vi "SC_schleife_init_20TVTI.vi"   [LabVIEW 2019]
uses:
  Monitors/Utility/Monitor Communication/Gustav/20TVTI_Control.ctl
  Global/Global Variables/global.vi
  Instrument_Setup.vi
  Global/Global Variables/Data_Display_global.vi
types:
  T1 = typedef "20TVTI_Cluster.ctl" = cluster{"Temperatur (K)":dbl, "Setpoint (K)":dbl, "Rate (K/min)":dbl, "Heater (%)":dbl, "NV (%)":dbl, "Heater Manual":bool, "NV Manual":bool, "Go to Set":bool, "Heater SP":dbl, "Valid?":bool, "Set Heater SP":bool, "Set NV SP":bool, "Heater (%) Display":dbl, "NV (%) Display":dbl, "NV Setpoint":dbl, "Change Heater Status":bool, "Change NV Status":bool, "Stop":bool, "Current T Setpoint":dbl, "Sweeping?":bool, "Sweep Mode":string, "Change Sweep Mode":bool}
  T2 = typedef "20TVTI_Control.ctl" = cluster{"Set VTI SP":bool, "Change NV Status":bool, "Set NV Setpoint":bool, "Change Heater Status":bool, "Set Heater Setpoint":bool, "Stop Sweep":bool, "Setpoint (K)":dbl, "Rate (K/min)":dbl, "Setpoint Heater":dbl, "Setpoint NV":dbl, "Change Sweep Mode":bool}
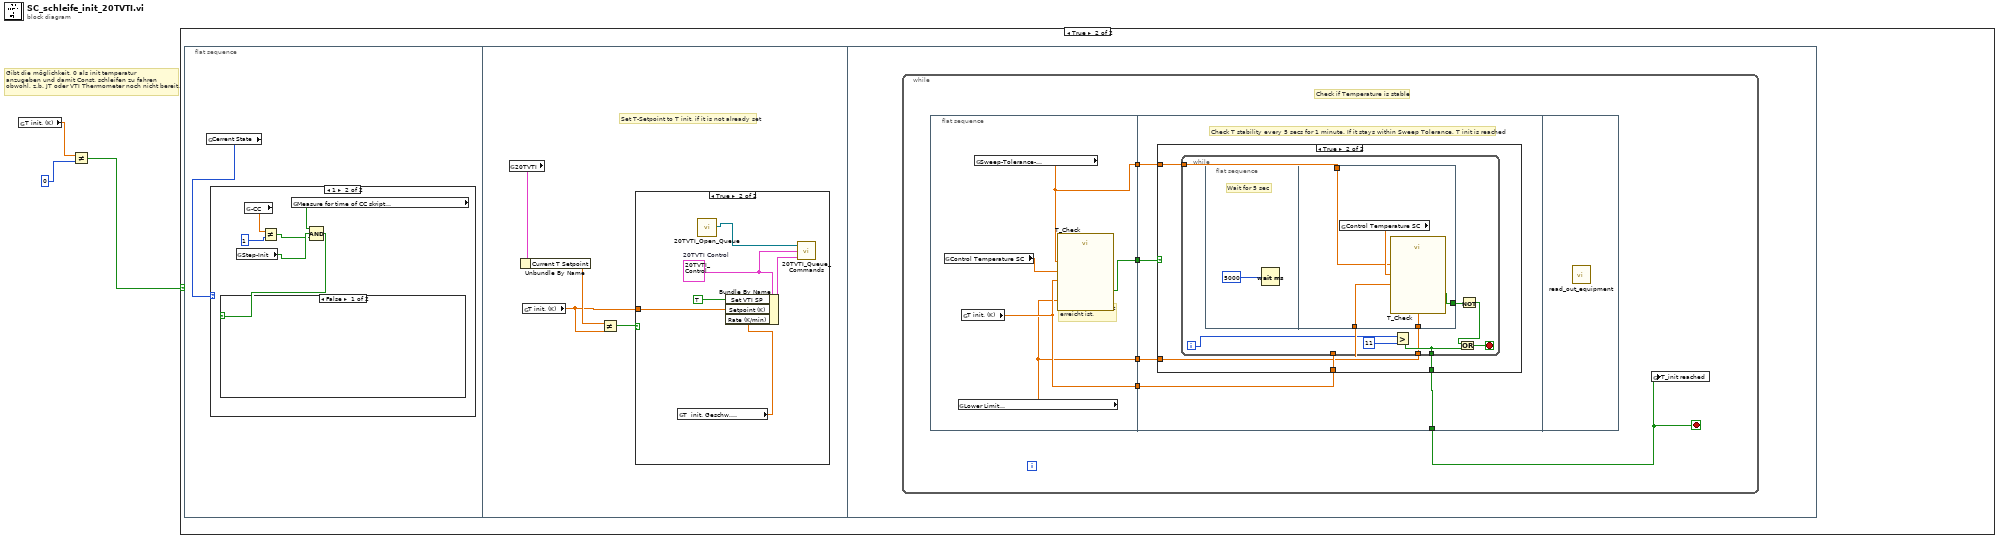
[diagram p0: block diagram]
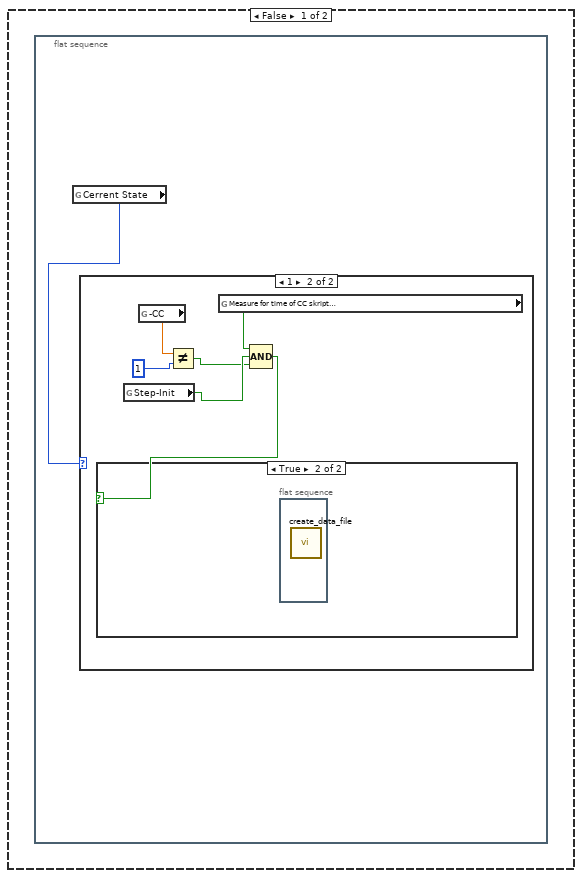
[diagram p2: hidden frame]
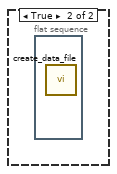
[diagram p6: hidden frame]
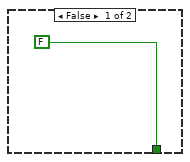
[diagram p8: hidden frame]
diagram:
  # "Gibt die möglichkeit, 0 als init temperatur \nanzugeben und damit Const. schleifen zu fahren\nobwohl, z.b. JT oder VTI Thermometer noch nicht bereit."
  n1 = global read "global.vi" "T init. (K)"() -> (w3:dbl)
  n2 = Not Equal?(x=w3, y=0) -> (x != y?=w1:bool)
  n3 = case shown="True" w1 {
    frame False {
      n4 = flat-sequence {
        frame #0 {
          n5 = global read "global.vi" "Cerrent State"() -> (w4:i32)
          n6 = case shown="1" w4 {
            frame 0, Default {
            }
            frame 1 {
              n7 = global read "global.vi" "Step-Init"() -> (w8:bool)
              n8 = global read "global.vi" "-CC"() -> (w7:dbl)
              n9 = Not Equal?(x=w7, y=1) -> (x != y?=w5:bool)
              n10 = global read "Instrument_Setup.vi" "Measure for time of CC skript\nat each field step point"() -> (w10:bool)
              n11 = Compound Arithmetic op=AND(w10, w8, w5) -> (w9:bool)
              n12 = case shown="True" w9 {
                frame False {
                }
                frame True {
                  n13 = flat-sequence {
                    frame #0 {
                      n14 = call "create_data_file.vi"() -> ()  [unwired: 3 in]
                    }
                  }
                }
              }
            }
          }
        }
      }
    }
    frame True {
      n15 = flat-sequence {
        frame #0 {
          n16 = global read "global.vi" "Cerrent State"() -> (w11:i32)
          n17 = case shown="1" w11 {
            frame 0, Default {
            }
            frame 1 {
              n18 = global read "global.vi" "Step-Init"() -> (w15:bool)
              n19 = global read "global.vi" "-CC"() -> (w14:dbl)
              n20 = Not Equal?(x=w14, y=1) -> (x != y?=w12:bool)
              n21 = global read "Instrument_Setup.vi" "Measure for time of CC skript\nat each field step point"() -> (w17:bool)
              n22 = Compound Arithmetic op=AND(w17, w15, w12) -> (w16:bool)
              n23 = case shown="False" w16 {
                frame False {
                }
                frame True {
                  n24 = flat-sequence {
                    frame #0 {
                      n25 = call "create_data_file.vi"() -> ()  [unwired: 3 in]
                    }
                  }
                }
              }
            }
          }
        }
        frame #1 {
          # "Set T-Setpoint to T init, if it is not already set"
          n26 = global read "Data_Display_global.vi" "20TVTI"() -> (w21:T1)
          n27 = Unbundle By Name(w21) -> ("Current T Setpoint"=w19:dbl)
          n28 = global read "global.vi" "T init. (K)"() -> (w18:dbl)
          n29 = Not Equal?(x=w19, y=w18) -> (x != y?=w20:bool)
          n30 = case shown="True" w20 {
            tunnel: w18 -> [_ w26]
            frame False {
            }
            frame True {
              w22 = T2 {"Set VTI SP"=FALSE, "Change NV Status"=FALSE, "Set NV Setpoint"=FALSE, "Change Heater Status"=FALSE, "Set Heater Setpoint"=FALSE, "Stop Sweep"=FALSE, "Setpoint (K)"=0.0, "Rate (K/min)"=0.0, "Setpoint Heater"=0.0, "Setpoint NV"=0.0, "Change Sweep Mode"=FALSE}  # 20TVTI Control
              n31 = global read "global.vi" "T  init. Geschw. \n(K/min)"() -> (w25:dbl)
              n32 = call "20TVTI_Open_Queue.vi"() -> ("queue out"=w24:refnum<queue>)  [unwired: 10 in, 1 out]
              n33 = Bundle By Name(cluster=w22, "Set VTI SP"=TRUE, "Setpoint (K)"=w26, "Rate (K/min)"=w25) -> (w23:T2)
              n34 = call "20TVTI_Queue_Commands.vi"("20TVTI Control"=w23, "Last Status"=w22, "20TVTI Queue"=w24) -> ()  [unwired: 1 out]
            }
          }
        }
        frame #2 {
          n35 = while {
            stop <- w32 stop-if-true
            # "Check if Temperature is stable"
            n36 = flat-sequence {
              tunnel: [w36] -> w31
              tunnel: [w35] -> w30
              tunnel: [w34] -> w29
              tunnel: [w33] -> w28
              tunnel: [w39] -> w32
              tunnel: w31 -> [w42]
              tunnel: w30 -> [w41]
              tunnel: w29 -> [w40]
              tunnel: w28 -> [w38]
              frame #0 {
                # "Check ob T_target\nerreicht ist."
                n37 = global read "Data_Display_global.vi" "Control Temperature SC"() -> (w37:dbl)
                n38 = global read "Instrument_Setup.vi" "Lower Limit\nSweep-Tolerance-\nTemperature (K)"() -> (w33:dbl)
                n39 = global read "global.vi" "T init. (K)"() -> (w35:dbl)
                n40 = global read "Instrument_Setup.vi" "Sweep-Tolerance-\nTemperature (%)"() -> (w34:dbl)
                n41 = call "T_Check.vi"("Lower Limit Sweep\nTolerance (K)"=w33, "T_target (K)"=w35, "Sweep\nTolerance %"=w34, "T_in"=w37) -> ("= T target"=w36:bool)
              }
              frame #1 {
                # "Check T stability every 5 secs for 1 minute. If it stays within Sweep Tolerance, T init is reached"
                n42 = case shown="True" w42 {
                  tunnel: w41 -> [_ w47]
                  tunnel: w40 -> [_ w46]
                  tunnel: [FALSE w45] -> w39
                  tunnel: w38 -> [_ w44]
                  frame False {
                  }
                  frame True {
                    n43 = while {
                      tunnel: w47 -> [w56]
                      tunnel: w46 -> [w55]
                      tunnel: [w49] -> w45
                      tunnel: w44 -> [w48]
                      i -> [w52]
                      stop <- w53 stop-if-true
                      n44 = flat-sequence {
                        tunnel: [w61] -> w54
                        tunnel: w56 -> [w60]
                        tunnel: w55 -> [w59]
                        tunnel: w48 -> [w58]
                        frame #0 {
                          # "Wait for 5 sec"
                          n45 = Wait (ms)(milliseconds to wait=5000) -> ()  [unwired: 1 out]
                        }
                        frame #1 {
                          n46 = global read "Data_Display_global.vi" "Control Temperature SC"() -> (w62:dbl)
                          n47 = call "T_Check.vi"("Lower Limit Sweep\nTolerance (K)"=w58, "T_target (K)"=w60, "Sweep\nTolerance %"=w59, "T_in"=w62) -> ("= T target"=w61:bool)
                        }
                      }
                      n48 = Greater?(x=w52, y=11) -> (0:w49:bool)
                      n49 = Not(x=w54) -> (.not. x?=w50:bool)
                      n50 = Or(x=w50, y=w49) -> (x .or. y?=w53:bool)
                    }
                  }
                }
              }
              frame #2 {
                n51 = call "read_out_equipment.vi"() -> ()  [unwired: 1 in]
              }
            }
            n52 = global write "Data_Display_global.vi" "T_init reached"(w32) -> ()
          }
        }
      }
    }
  }
